vi "Global Configration.vi"(2 "Error In":errorcluster, 3 "Action":T1, 4 "Parameters In":T2 {"RunType" items=["Diagnostics", "Tune", "Acquisition"]}) -> (0 "Error Out":errorcluster, 1 "Parameters Out":T2 {"RunType" items=["Diagnostics", "Tune", "Acquisition"]})   [LabVIEW 2018]
uses:
  Type Defs/Global Configrations.ctl
  Type Defs/Configration.ctl
  GC-MSMSDevlopment/Type/_RT Configuration 2.ctl
  Type Defs/ADC Table.ctl
  Type Defs/Global Action.ctl
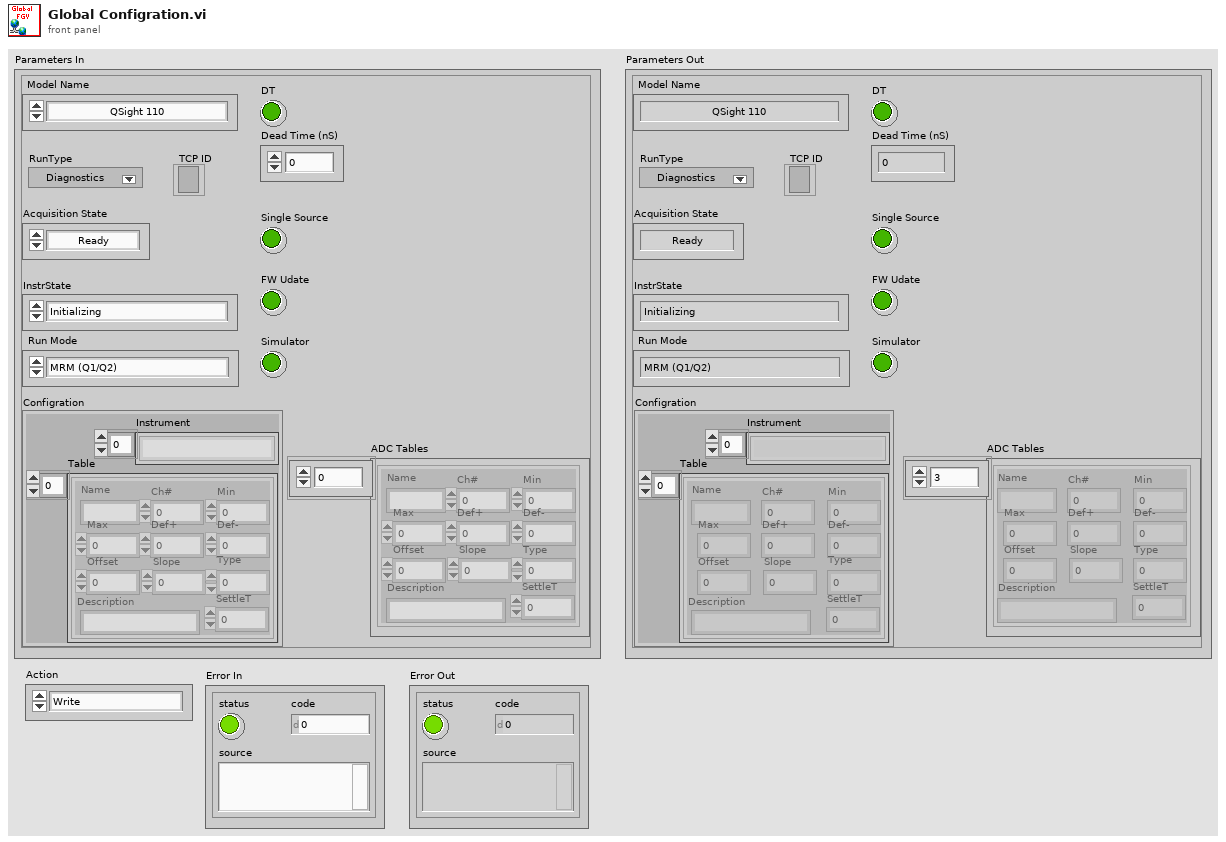
[diagram p1: front panel]
types:
  T1 = typedef "Global Action.ctl" = enum16{"Write", "Read"}
  T2 = typedef "Global Configrations.ctl" = cluster{"Model Name":enum16{"QSight 110", "QSight 120", "QSight 210", "QSight 220", "QSight 410", "QSight 420", "IONICS 3Q 110", "IONICS 3Q 120", "IONICS 3Q 210", "IONICS 3Q 220", "IONICS 3Q 310", "IONICS 3Q 320", "Simulation (Single Source)", "Simulation (Dual Source)"}, "RunType":u16, "Acquisition State":enum16{"Ready", "Busy", "Waiting"}, "InstrState":enum16{"Initializing", "Mass Spectrometer is Off", "Starting Up", "Turning Power Off", "Going to Standby", "Roughing Pump Ready", "Turning Turbo Off", "Turbo Startup", "Turbopump Ready", "Checking Vacuum", "Going to Ready", "Ready", "Running", "Source Standby", "Lost Communication", "Shutting Down", "Fault", "24V Standby", "Go to 24V Standby", "Turbopump Ready-Waiting"}, "Run Mode":enum16{"MRM (Q1/Q2)", "Q1 Scan", "Q1 SRM", "Q2 Scan", "Q2 SRM", "Product Scan", "Precursor Scan", "Neutral Loss", "Neutral Gain"}, "Configration":T3, "TCP ID":refnum<k5>, "DT":bool, "Dead Time (nS)":i32, "Single Source":bool, "ADC Tables":T5[], "FW Udate":bool, "Simulator":bool}
  T3 = typedef "Configration.ctl" = cluster{"Table":T4[], "Instrument":string[]}
  T4 = typedef "_RT Configuration 2.ctl" = cluster{"Name":string, "Ch#":u8, "Min":dbl, "Max":dbl, "Def+":dbl, "Def-":dbl, "Offset":dbl, "Slope":dbl, "Type":u8, "Description":string, "SettleT":dbl}
  T5 = typedef "ADC Table.ctl" = cluster{"Name":string, "Ch#":u8, "Min":dbl, "Max":dbl, "Def+":dbl, "Def-":dbl, "Offset":dbl, "Slope":dbl, "Type":u8, "Description":string, "SettleT":dbl}
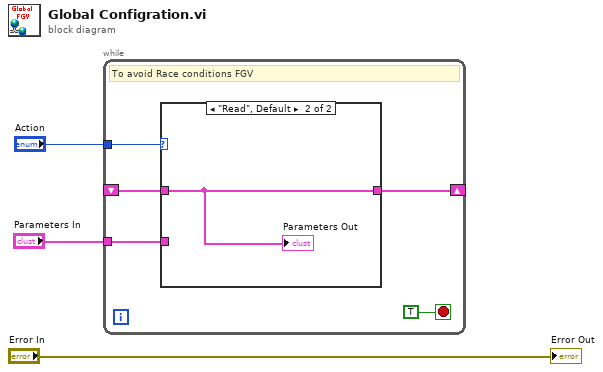
[diagram p0: block diagram]
diagram:
  n1 = while {
    shift-right: [w5] -> _
    shift-left: _ -> [w6]
    tunnel: "Action" -> [w7]
    tunnel: "Parameters In" -> [w4]
    stop <- TRUE stop-if-true
    # "To avoid Race conditions FGV"
    n2 = case shown="\"Read\", Default" w7 {
      tunnel: w6 -> [_ w10]
      tunnel: [w9 w10] -> w5
      tunnel: w4 -> [w9 _]
      frame "Write" {
      }
      frame "Read", Default {
        "Parameters Out" <- w10
      }
    }
  }
  "Error Out" <- "Error In"
